vi "ryTimer Daemon.vi"(4 "Ignore if exists?":bool, 6 "One Shot?":bool, 7 "Callback Custom":refnum<vi>, 8 "Message":string, 9 "Destination Refnum":string, 10 "Callback Type":enum8{"Queue", "UserEvent", "Custom"}(ring), 11 "Properties":refnum<data-value>) -> ()   [LabVIEW 2020, in "ryTimer.lvclass"]
uses:
  ryTimer.lvclass
  TypeDefs/ryTimer Properties.ctl
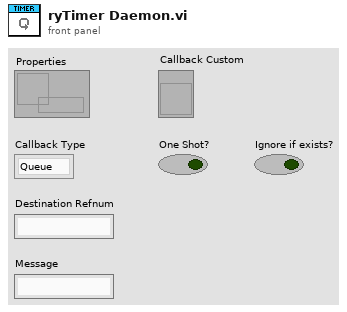
[diagram p1: front panel]
types:
  T1 = typedef "ryTimer.lvclass/ryTimer Properties.ctl" = cluster{"Wait Time (ms)":u32, "Is Running":bool, "Last Ticks":u32, "Emit":refnum<queue>}
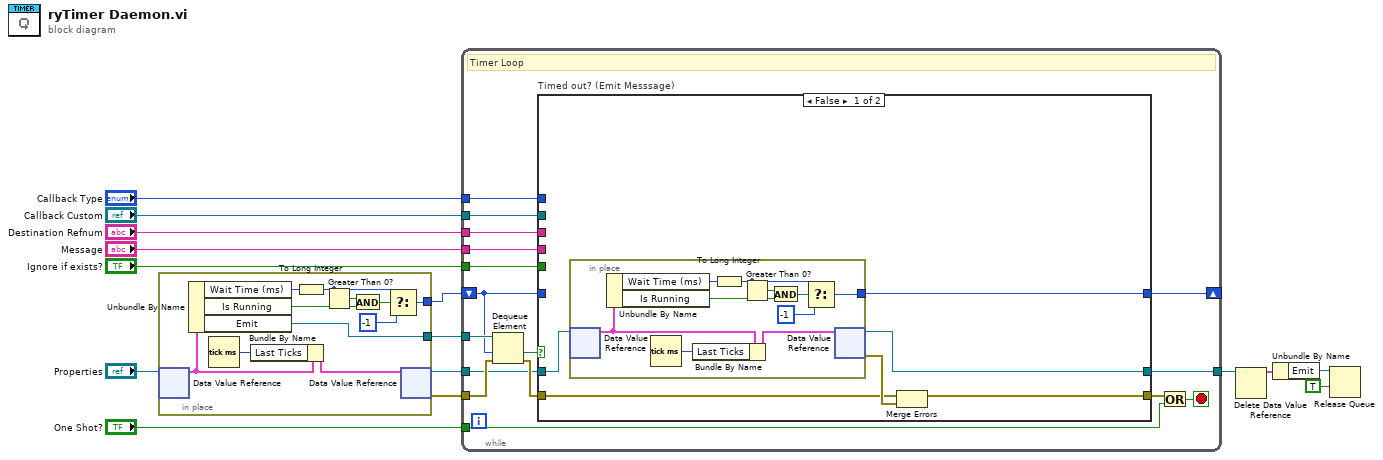
[diagram p0: block diagram]
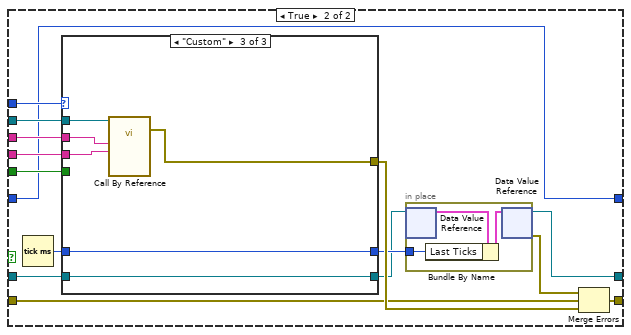
[diagram p2: hidden frame]
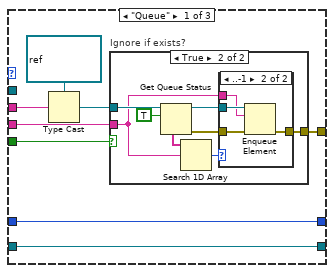
[diagram p3: hidden frame]
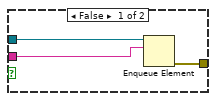
[diagram p4: hidden frame]
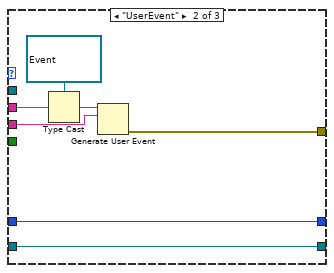
[diagram p6: hidden frame]
diagram:
  n1 = in-place {
    in-place-border: [w20] -> w7
    in-place-border: [w19] -> w6
    n2 = in-place-dvr #1("Properties") -> (w18:T1)  [unwired: 1 out]
    n3 = Unbundle By Name(w18) -> ("Wait Time (ms)"=w22:u32, "Is Running"=w26:bool, "Emit"=w19:refnum<queue>)
    n4 = Tick Count (ms)() -> (millisecond timer value=w16:u32)
    n5 = Bundle By Name(cluster=w18, "Last Ticks"=w16) -> (w17:T1)
    n6 = To Long Integer(number=w22) -> (32bit integer=w23:i32)
    n7 = Greater Than 0?(x=w23) -> (x > 0?=w24:bool)
    n8 = And(x=w24, y=w26) -> (x .and. y?=w25:bool)
    n9 = Select(t=w23, s=w25, f=-1 ("timeout in ms (-1)")) -> (s? t:f=w20:i32)
    n10 = in-place-dvr #1(w17) -> (w2:refnum<data-value>, w1:errorcluster)
  }
  n11 = while {
    tunnel: w2 -> [w29]
    tunnel: "One Shot?" -> [w42]
    tunnel: "Callback Type" -> [w38]
    tunnel: "Destination Refnum" -> [w37]
    tunnel: "Message" -> [w36]
    tunnel: "Callback Custom" -> [w35]
    tunnel: [w33] -> w5
    tunnel: "Ignore if exists?" -> [w32]
    shift-right: [w27] -> _
    shift-left: w7 -> [w28]
    tunnel: w1 -> [w31]
    tunnel: w6 -> [w30]
    stop <- w41 stop-if-true
    # "Timer Loop"
    n12 = Dequeue Element(queue=w30, timeout in ms (-1)=w28, error in (no error)=w31) -> (timed out?=w39:bool, error out=w34:errorcluster)  [unwired: 2 out]
    n13 = case "Timed out? (Emit Messsage)" shown="False" w39 {
      tunnel: [w45 w68] -> w40
      tunnel: w29 -> [w47 w70]
      tunnel: w38 -> [_ w73]
      tunnel: w37 -> [_ w72]
      tunnel: w36 -> [_ w71]
      tunnel: w35 -> [_ w66]
      tunnel: w34 -> [w44 w60]
      tunnel: [w43 w59] -> w33
      tunnel: w32 -> [_ w65]
      tunnel: w28 -> [_ w63]
      tunnel: [w48 w63] -> w27
      frame False {
        n14 = in-place {
          in-place-border: [w53] -> w48
          n15 = in-place-dvr #2(w47) -> (w51:T1)  [unwired: 1 out]
          n16 = Unbundle By Name(w51) -> ("Wait Time (ms)"=w57:u32, "Is Running"=w52:bool)
          n17 = Tick Count (ms)() -> (millisecond timer value=w49:u32)
          n18 = Bundle By Name(cluster=w51, "Last Ticks"=w49) -> (w50:T1)
          n19 = To Long Integer(number=w57) -> (32bit integer=w56:i32)
          n20 = Greater Than 0?(x=w56) -> (x > 0?=w55:bool)
          n21 = And(x=w55, y=w52) -> (x .and. y?=w54:bool)
          n22 = Select(t=w56, s=w54, f=-1 ("timeout in ms (-1)")) -> (s? t:f=w53:i32)
          n23 = in-place-dvr #2(w50) -> (w43:refnum<data-value>, w46:errorcluster)
        }
        n24 = Merge Errors(w44, w46) -> (w45:errorcluster)
      }
      frame True {
        n25 = Tick Count (ms)() -> (millisecond timer value=w69:u32)
        n26 = case shown="\"Custom\"" w73 {
          tunnel: w72 -> [w84 w107 w110]
          tunnel: w71 -> [w78 w105 w109]
          tunnel: [w82 w104 w113] -> w67
          tunnel: [w80 w102 w108] -> w62
          tunnel: w70 -> [w80 w102 w108]
          tunnel: w69 -> [w81 w101 w111]
          tunnel: [w81 w101 w111] -> w64
          tunnel: w66 -> [_ _ w112]
          tunnel: w65 -> [w77 _ _]
          frame "Queue" {
            n27 = Type Cast(type=refnum<queue> refnum ("Queue"), x=w84) -> (*(type *) &x=w79:refnum<queue>)
            n28 = case "Ignore if exists?" shown="True" w77 {
              tunnel: [w85 w95] -> w82
              tunnel: w79 -> [w87 w94]
              tunnel: w78 -> [w86 w91]
              frame False {
                n29 = Enqueue Element(queue=w87, element=w86) -> (error out=w85:errorcluster)  [unwired: 2 in, 2 out]
              }
              frame True {
                n30 = Get Queue Status(queue=w94, return elements? (F)=TRUE) -> (queue out=w93:refnum<queue>, error out=w89:errorcluster, elements=w92:string[])  [unwired: 1 in, 5 out]
                n31 = Search 1D Array(1D array=w92, element=w91) -> (index of element=w88:i32)  [unwired: 1 in]
                n32 = case shown="..-1" w88 {
                  tunnel: [w96 w100] -> w95
                  tunnel: w93 -> [_ w99]
                  tunnel: w91 -> [_ w98]
                  tunnel: w89 -> [w96 w97]
                  frame 0.. {
                  }
                  frame ..-1 {
                    n33 = Enqueue Element(queue=w99, element=w98, error in (no error)=w97) -> (error out=w100:errorcluster)  [unwired: 1 in, 2 out]
                  }
                }
              }
            }
          }
          frame "UserEvent" {
            n34 = Type Cast(type=refnum<user-event> refnum ("User Event"), x=w107) -> (*(type *) &x=w106:refnum<user-event>)
            n35 = Generate User Event(user event=w106, event data cluster=w105) -> (error out=w104:errorcluster)  [unwired: 2 in, 1 out]
          }
          frame "Custom" {
            n36 = call-by-ref "?"(reference=w112, "Message"=w109, "Destination Refnum"=w110) -> (error out=w113:errorcluster)  [unwired: 11 in, 1 out]
          }
        }
        n37 = in-place {
          in-place-border: w64 -> [w76]
          n38 = in-place-dvr #3(w62) -> (w75:T1)  [unwired: 1 out]
          n39 = Bundle By Name(cluster=w75, "Last Ticks"=w76) -> (w74:T1)
          n40 = in-place-dvr #3(w74) -> (w59:refnum<data-value>, w61:errorcluster)
        }
        n41 = Merge Errors(w61, w60, w67) -> (w68:errorcluster)
      }
    }
    n42 = Or(x=w40, y=w42) -> (x .or. y?=w41:bool)
  }
  n43 = Delete Data Value Reference(data value reference=w5) -> (data value=w4:T1)  [unwired: 1 in, 1 out]
  n44 = Unbundle By Name(w4) -> ("Emit"=w10:refnum<queue>)
  n45 = Release Queue(queue=w10, force destroy? (F)=TRUE) -> ()  [unwired: 1 in, 3 out]
